vi "Write Background Control Queue.vi"(8 "error in (no error)":errorcluster, 10 "Background Control Queue":refnum<queue>, 11 "Socket in":refnum<class "Execution.lvclass">) -> (0 "error out":errorcluster, 3 "Socket out":refnum<class "Execution.lvclass">)   [LabVIEW 2015, in "Execution.lvclass"]
uses:
  Execution.lvclass
  BACKGROUND_CONTROL_MSG_TYPEDEF.ctl
  Execution.lvclass/Execution.ctl
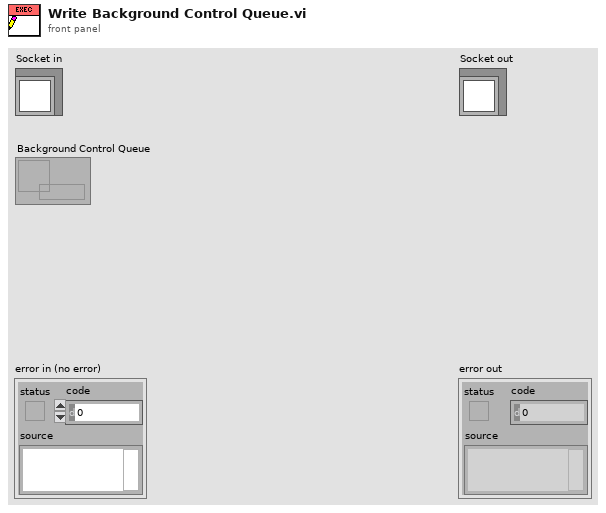
[diagram p1: front panel]
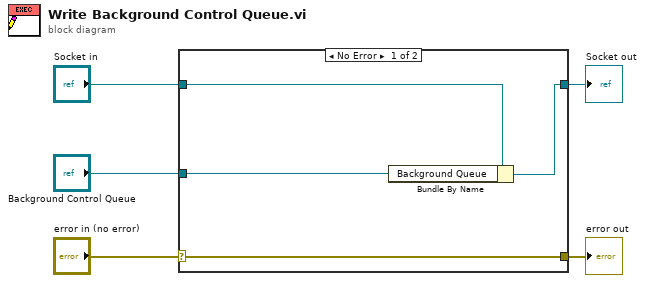
[diagram p0: block diagram]
diagram:
  n1 = case shown="No Error" "error in (no error)" {
    selector: "error in (no error)" -> [w9 w10]
    tunnel: [w9 w10] -> w4
    tunnel: [w7 w11] -> w2
    tunnel: "Socket in" -> [w8 w11]
    tunnel: "Background Control Queue" -> [w6 _]
    frame No Error {
      n2 = Bundle By Name(cluster=w8, "Background Queue"=w6) -> (w7:refnum<class "Execution.lvclass">)
    }
    frame Error {
    }
  }
  "error out" <- w4
  "Socket out" <- w2
